vi "CAlex2_SetCuff_Thigh.vi"(6 "Knee Distance Reference":T1(ring), 9 "ExtraWeight":dbl, 10 "Thigh Cuff Low Distance From Bottom (Hole*0.00635)":dbl, 11 "Knee Distance":dbl) -> (2 "Thigh Cuff Low":T2={"BodyID"=0, "CoM(CuffCS)"={"Coord4"=[0.0, 0.0, 0.0, 1.0], "ID"=0}, "Mass(kg)"=0.0, "CablePts(CuffCS)"=[], "Cuff->Body"=[[1.0, 0.0, 0.0, 0.0], [0.0, 1.0, 0.0, 0.0], [0.0, 0.0, 1.0, 0.0], [0.0, 0.0, 0.0, 1.0]]}, 3 "Thigh Cuff High":T2={"BodyID"=0, "CoM(CuffCS)"={"Coord4"=[0.0, 0.0, 0.0, 1.0], "ID"=0}, "Mass(kg)"=0.0, "CablePts(CuffCS)"=[], "Cuff->Body"=[[1.0, 0.0, 0.0, 0.0], [0.0, 1.0, 0.0, 0.0], [0.0, 0.0, 1.0, 0.0], [0.0, 0.0, 0.0, 1.0]]} {"CoM(CuffCS)"."Coord4" format="%#_6f"})   [LabVIEW 2015, in "CAlex2.lvclass"]
uses:
  CAlex2.lvclass
  CableSerialChain/TypeDef/Cuff.ctl
  Body/PointOnBody.ctl
  <vilib>/Analysis/Matrix/Datatypes/RealMatrix.ctl
  <vilib>/Analysis/Matrix/NI_Matrix.lvlib
  Body/Bodies.lvclass
  CableSerialChain/CableSerialChain.lvclass
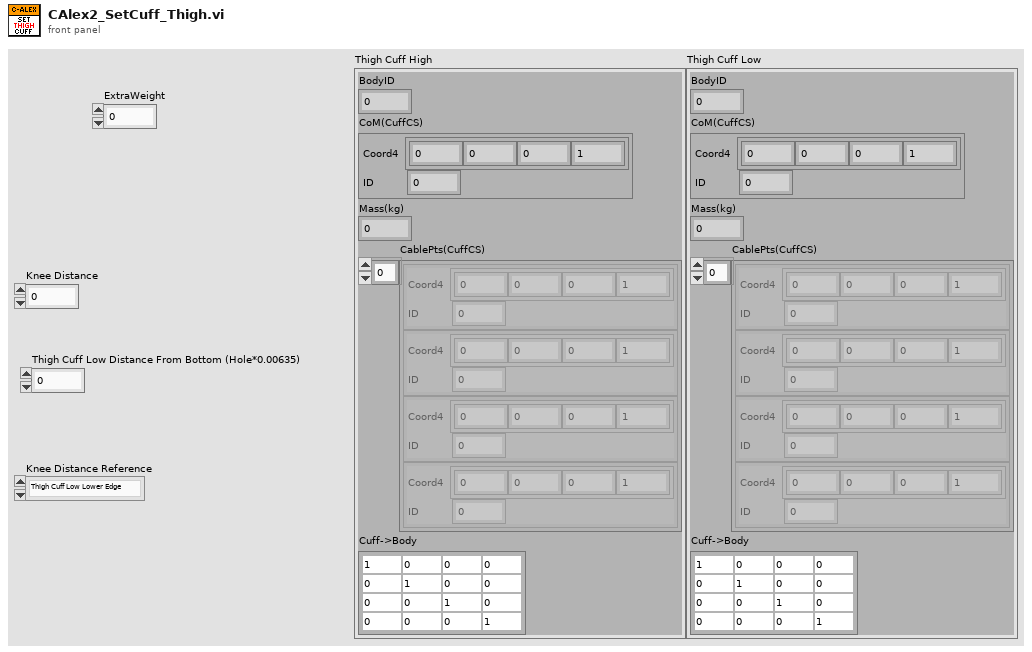
[diagram p1: front panel]
types:
  T1 = enum16{"Thigh Cuff Low Lower Edge", "Thigh Cuff High Center"}
  T2 = typedef "CableSerialChain.lvclass/Cuff.ctl" = cluster{"BodyID":i32, "CoM(CuffCS)":T3, "Mass(kg)":dbl, "CablePts(CuffCS)":T3[], "Cuff->Body":T4}
  T3 = typedef "Bodies.lvclass/PointOnBody.ctl" = cluster{"Coord4":dbl[], "ID":i32}
  T4 = typedef "NI_Matrix.lvlib/RealMatrix.ctl" = dbl[][]
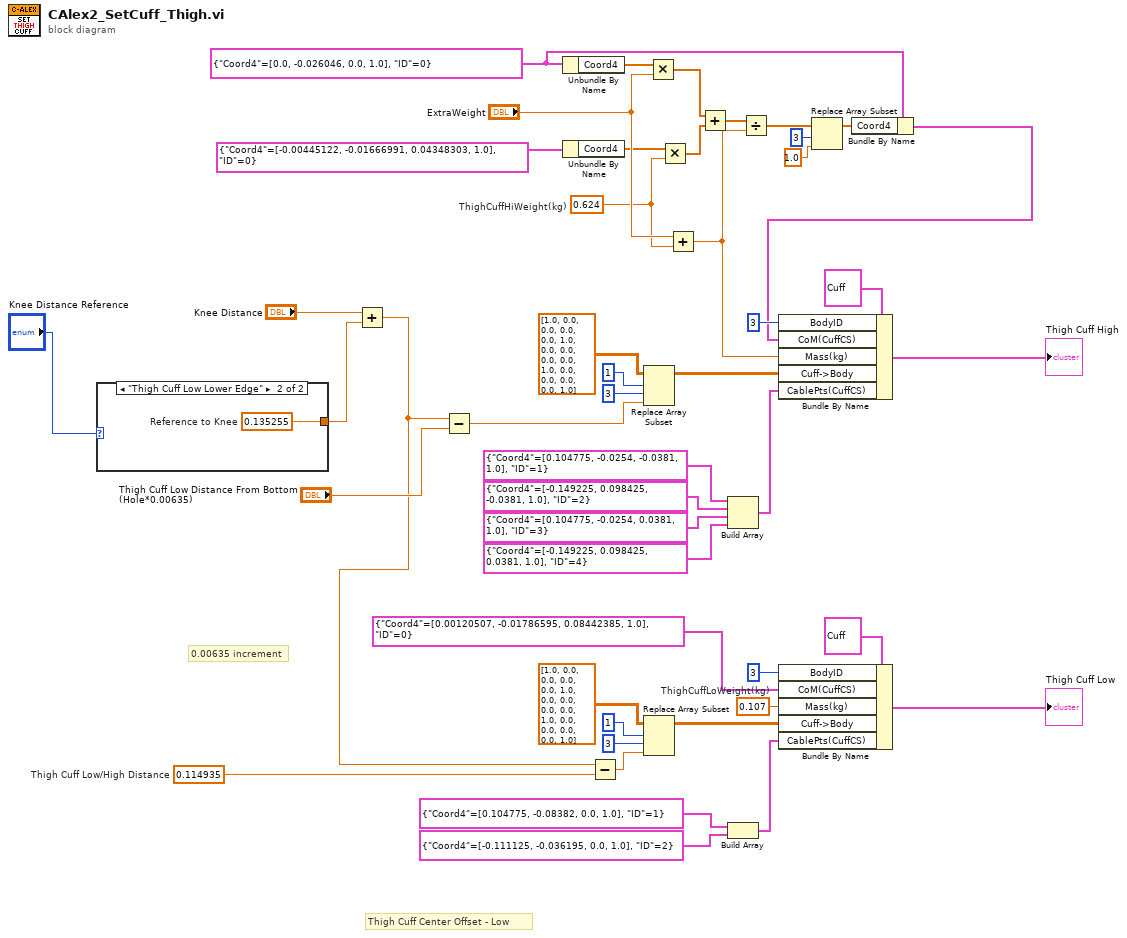
[diagram p0: block diagram]
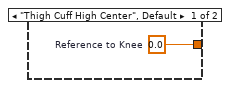
[diagram p2: hidden frame]
diagram:
  w10 = T3 {"Coord4"=[0.0, -0.026046, 0.0, 1.0], "ID"=0} ("CoM(CuffCS)")
  w2 = 0.114935  # Thigh Cuff Low/High Distance
  w25 = 0.107  # ThighCuffLoWeight(kg)
  w15 = 0.624  # ThighCuffHiWeight(kg)
  # "0.00635 increment"
  # "Thigh Cuff Center Offset - Low"
  n1 = case shown="\"Thigh Cuff Low Lower Edge\"" "Knee Distance Reference" {
    tunnel: [w48 w49] -> w35
    frame "Thigh Cuff High Center", Default {
      w48 = 0.0  # Reference to Knee
    }
    frame "Thigh Cuff Low Lower Edge" {
      w49 = 0.135255  # Reference to Knee
    }
  }
  n2 = Add(x="Knee Distance", y=w35) -> (x+y=w1:dbl)
  n3 = Subtract(x=w1, y="Thigh Cuff Low Distance From Bottom (Hole*0.00635)") -> (x-y=w4:dbl)
  n4 = Unbundle By Name(w10) -> ("Coord4"=w18:dbl[])
  n5 = Unbundle By Name(T3 {"Coord4"=[-0.00445122, -0.01666991, 0.04348303, 1.0], "ID"=0} ("CoM(CuffCS)")) -> ("Coord4"=w16:dbl[])
  n6 = Subtract(x=w1, y=w2) -> (x-y=w34:dbl)
  n7 = Replace Array Subset(array=T4 [[1.0, 0.0, 0.0, 0.0], [0.0, 1.0, 0.0, 0.0], [0.0, 0.0, 1.0, 0.0], [0.0, 0.0, 0.0, 1.0]] ("Cuff->Leg"), new element=w4, index (row)=1, index (col)=3 ("index (row)")) -> (w44:T4)
  n8 = Replace Array Subset(array=T4 [[1.0, 0.0, 0.0, 0.0], [0.0, 1.0, 0.0, 0.0], [0.0, 0.0, 1.0, 0.0], [0.0, 0.0, 0.0, 1.0]] ("Cuff->Leg"), new element=w34, index (row)=1, index (col)=3 ("index (row)")) -> (w27:T4)
  n9 = Multiply(x=w18, y="ExtraWeight") -> (x*y=w14:dbl[])
  n10 = Multiply(x=w16, y=w15) -> (x*y=w13:dbl[])
  n11 = Add(x="ExtraWeight", y=w15) -> (x+y=w11:dbl)
  n12 = Add(x=w14, y=w13) -> (x+y=w12:dbl[])
  n13 = Build Array(T3 {"Coord4"=[0.104775, -0.0254, -0.0381, 1.0], "ID"=1} ("CoM(CuffCS)"), T3 {"Coord4"=[-0.149225, 0.098425, -0.0381, 1.0], "ID"=2} ("CoM(CuffCS)"), T3 {"Coord4"=[0.104775, -0.0254, 0.0381, 1.0], "ID"=3} ("CoM(CuffCS)"), T3 {"Coord4"=[-0.149225, 0.098425, 0.0381, 1.0], "ID"=4} ("CoM(CuffCS)")) -> (w41:T3[])
  n14 = Build Array(T3 {"Coord4"=[0.104775, -0.08382, 0.0, 1.0], "ID"=1} ("CoM(CuffCS)"), T3 {"Coord4"=[-0.111125, -0.036195, 0.0, 1.0], "ID"=2} ("CoM(CuffCS)")) -> (w28:T3[])
  n15 = Divide(x=w12, y=w11) -> (x/y=w8:dbl[])
  n16 = Bundle By Name(cluster=T2 {"BodyID"=0, "CoM(CuffCS)"={"Coord4"=[0.0, 0.0, 0.0, 1.0], "ID"=0}, "Mass(kg)"=0.0, "CablePts(CuffCS)"=[], "Cuff->Body"=[[1.0, 0.0, 0.0, 0.0], [0.0, 1.0, 0.0, 0.0], [0.0, 0.0, 1.0, 0.0], [0.0, 0.0, 0.0, 1.0]]} ("Cuff Design"), "BodyID"=3, "CoM(CuffCS)"=T3 {"Coord4"=[0.00120507, -0.01786595, 0.08442385, 1.0], "ID"=0}, "Mass(kg)"=w25, "Cuff->Body"=w27, "CablePts(CuffCS)"=w28) -> (→"Thigh Cuff Low":T2)
  n17 = Replace Array Subset(array=w8, new element=1.0 ("new element/subarray"), index=3) -> (w7:dbl[])
  n18 = Bundle By Name(cluster=w10, "Coord4"=w7) -> (w9:T3)
  n19 = Bundle By Name(cluster=T2 {"BodyID"=0, "CoM(CuffCS)"={"Coord4"=[0.0, 0.0, 0.0, 1.0], "ID"=0}, "Mass(kg)"=0.0, "CablePts(CuffCS)"=[], "Cuff->Body"=[[1.0, 0.0, 0.0, 0.0], [0.0, 1.0, 0.0, 0.0], [0.0, 0.0, 1.0, 0.0], [0.0, 0.0, 0.0, 1.0]]} ("Cuff Design"), "BodyID"=3, "CoM(CuffCS)"=w9, "Mass(kg)"=w11, "Cuff->Body"=w44, "CablePts(CuffCS)"=w41) -> (→"Thigh Cuff High":T2)
